vi "BodyParser.vi"(8 "error in (no error)":errorcluster, 11 "body":string) -> (0 "error out":errorcluster, 2 "Array":cluster{"id":string, string}[](array[cluster]), 3 "Data array":T1(array[cluster]))   [LabVIEW 2019]
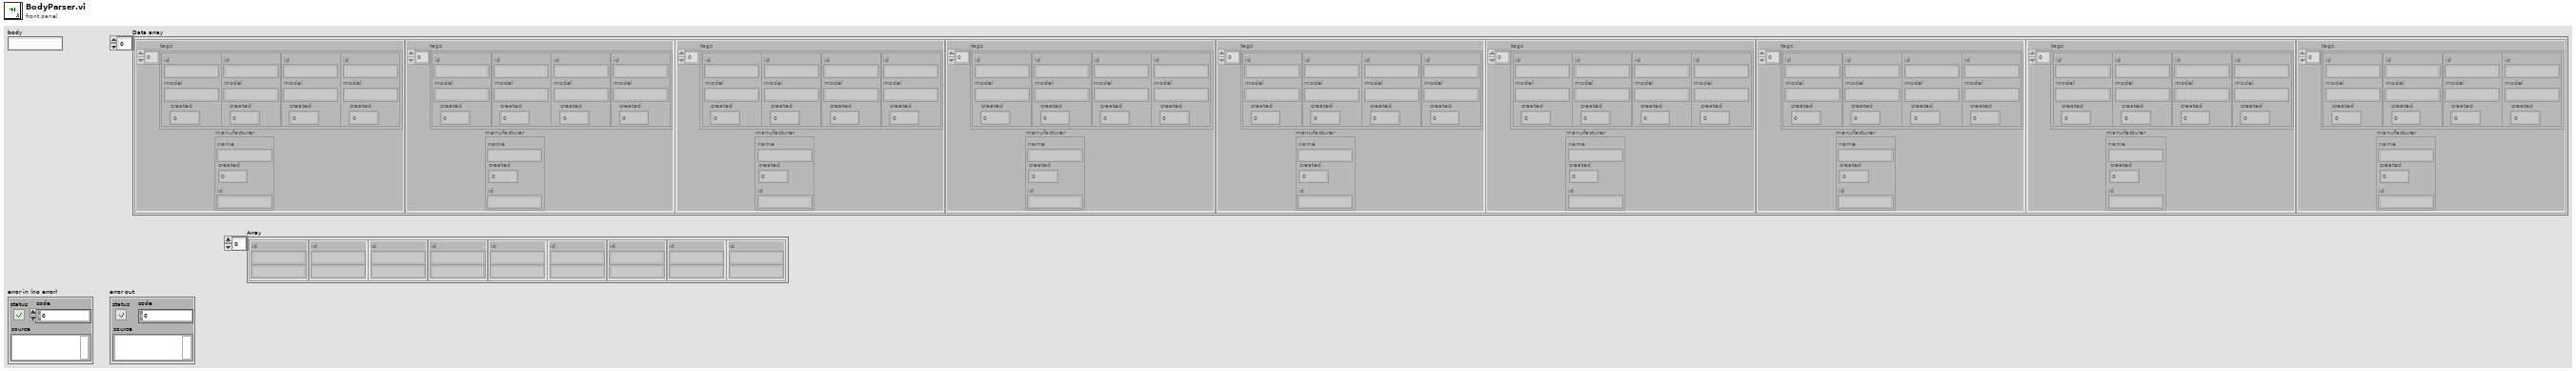
[diagram p1: front panel]
types:
  T1 = cluster{"tags":cluster{"id":string, "model":string, "created":i32}[], "manufacturer":cluster{"name":string, "created":i32, "id":string}}[]
  T2 = cluster{cluster{"tags":cluster{"id":string, "model":string, "created":i32}[], "manufacturer":cluster{"name":string, "created":i32, "id":string}}}[]
  T3 = cluster{cluster{"tags":cluster{"id":string, "model":string, "created":i32}[], "manufacturer":cluster{"name":string, "created":i32, "id":string}}}
  T4 = cluster{"tags":cluster{"id":string, "model":string, "created":i32}[], "manufacturer":cluster{"name":string, "created":i32, "id":string}}
  T5 = cluster{"id":string, "model":string, "created":i32}[]
  T6 = cluster{"name":string, "created":i32, "id":string}
  T7 = cluster{"id":string, "model":string, "created":i32}
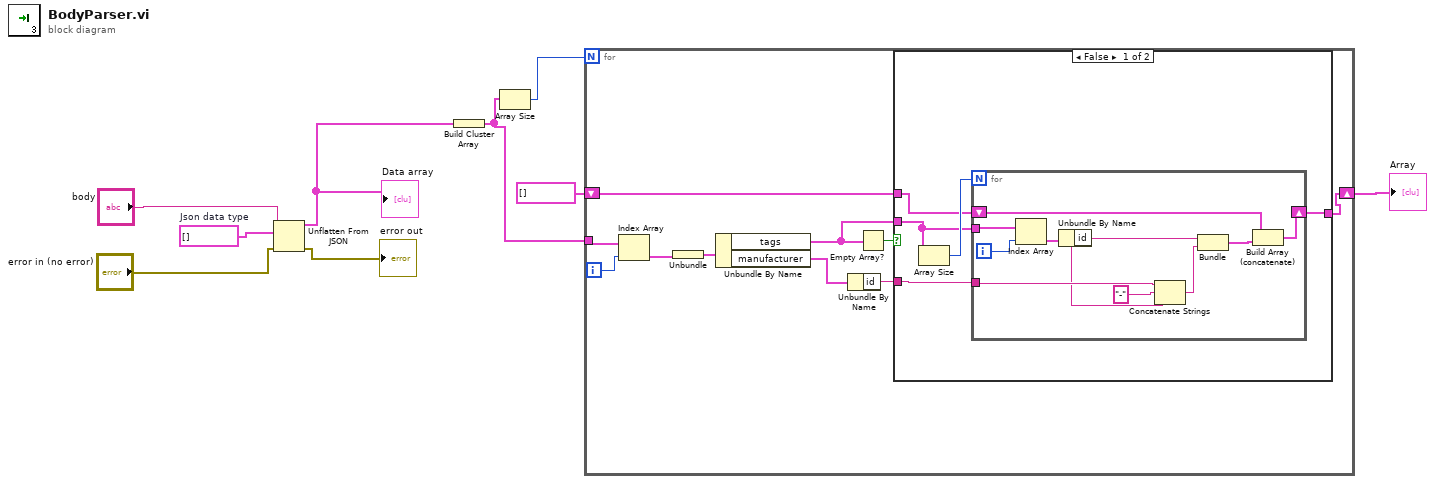
[diagram p0: block diagram]
diagram:
  w2 = T1 []  # Json data type
  n1 = Unflatten From JSON(JSON string="body", type and defaults=w2, error in (no error)="error in (no error)") -> (value=w4:T1, error out=→"error out":errorcluster)  [unwired: 4 in]
  "Data array" <- w4
  n2 = Build Cluster Array(w4) -> (w5:T2)
  n3 = Array Size(array=w5) -> (size(s)=w6:i32)
  n4 = for {
    N: w6 -> [_]
    tunnel: w5 -> [w17]
    shift-right: [w11] -> w7
    shift-left: cluster{"id":string, string}[] [] -> [w10]
    i -> [w16]
    n5 = Index Array(array=w17, index=w16) -> (element=w19:T3)
    n6 = Unbundle(w19) -> (w18:T4)
    n7 = Unbundle By Name(w18) -> ("tags"=w12:T5, "manufacturer"=w15:T6)
    n8 = Unbundle By Name(w15) -> ("id"=w13:string)
    n9 = Empty Array?(array=w12) -> (empty?=w14:bool)
    n10 = case shown="False" w14 {
      tunnel: w13 -> [w22 _]
      tunnel: w12 -> [w23 _]
      tunnel: [w21 w35] -> w11
      tunnel: w10 -> [w20 w35]
      frame False {
        n11 = Array Size(array=w23) -> (size(s)=w24:i32)
        n12 = for {
          N: w24 -> [_]
          tunnel: w23 -> [w33]
          tunnel: w22 -> [w31]
          shift-right: [w26] -> w21
          shift-left: w20 -> [w25]
          i -> [w34]
          n13 = Index Array(array=w33, index=w34) -> (element=w32:T7)
          n14 = Unbundle By Name(w32) -> ("id"=w29:string)
          n15 = Concatenate Strings(w31, "-" ("string"), w29) -> (w28:string)
          n16 = Bundle("id"=w29, w28) -> (w27:cluster{"id":string, string})  [unwired: 1 in]
          n17 = Build Array (concatenate)(w25, w27) -> (w26:cluster{"id":string, string}[])
        }
      }
      frame True {
      }
    }
  }
  "Array" <- w7
